vi "Limit Motion Values.vi"(11 "States In":T1 format="%.4f") -> (3 "States Out":T1 format="%.4f")   [LabVIEW 2018]
uses:
  States.ctl
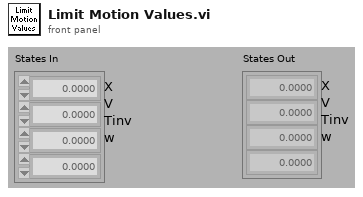
[diagram p1: front panel]
types:
  T1 = typedef "States.ctl" = dbl[]
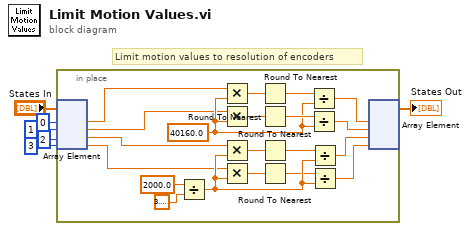
[diagram p0: block diagram]
diagram:
  # "Limit motion values to resolution of encoders"
  n1 = in-place {
    w17 = 40160.0 ("value")
    n2 = in-place-array #1("States In", 0, 1, 2, 3) -> (w14:dbl, w13:dbl, w12:dbl, w11:dbl)
    n3 = Divide(x=2000.0 ("value"), y=3.141592653589793) -> (x/y=w26:dbl)
    n4 = Multiply(x=w14, y=w17) -> (x*y=w15:dbl)
    n5 = Multiply(x=w13, y=w17) -> (x*y=w16:dbl)
    n6 = Multiply(x=w12, y=w26) -> (x*y=w23:dbl)
    n7 = Multiply(x=w11, y=w26) -> (x*y=w22:dbl)
    n8 = Round To Nearest(number=w15) -> (nearest integer value=w18:dbl)
    n9 = Round To Nearest(number=w16) -> (nearest integer value=w19:dbl)
    n10 = Round To Nearest(number=w23) -> (nearest integer value=w24:dbl)
    n11 = Round To Nearest(number=w22) -> (nearest integer value=w25:dbl)
    n12 = Divide(x=w18, y=w17) -> (x/y=w10:dbl)
    n13 = Divide(x=w19, y=w17) -> (x/y=w9:dbl)
    n14 = Divide(x=w24, y=w26) -> (x/y=w8:dbl)
    n15 = Divide(x=w25, y=w26) -> (x/y=w7:dbl)
    n16 = in-place-array #1(w10, w9, w8, w7) -> (→"States Out":T1)  [unwired: 4 out]
  }
